vi "Move Distance in Constant Acceleration.vi"(7 "Time Between Points (ms)":dbl, 8 "Error In":errorcluster, 9 "Acceleration (in/s2)":dbl, 10 "Distance (in)":dbl, 11 "Initial Snapshot":T2) -> (0 "Error Out":errorcluster, 1 "Duration (s)":dbl, 2 "Motion Profile Portion":T1[](array[typedef]), 3 "Final Snapshot":T2)   [LabVIEW 2019, in "Motion Profile Generator.lvclass"]
uses:
  Motion Profile Generator.lvclass
  Type Defs/Motion Snapshot.ctl
  Type Defs/Motion Profile Point.ctl
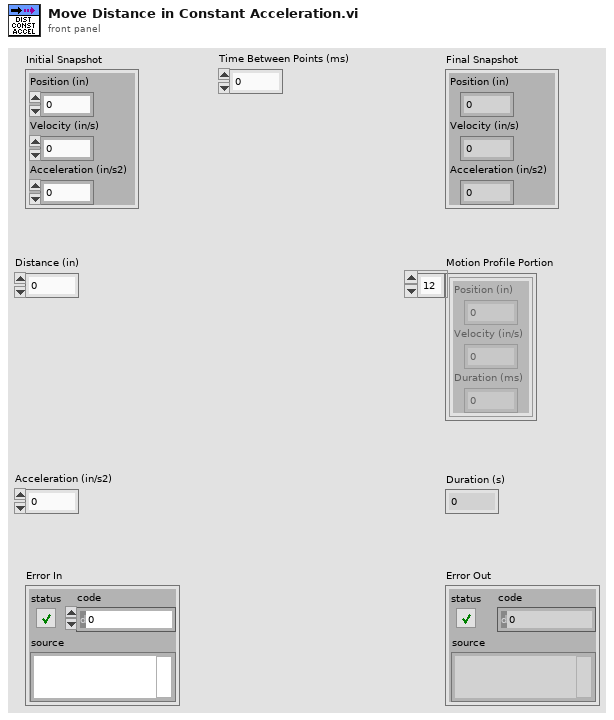
[diagram p1: front panel]
types:
  T1 = typedef "Motion Profile Generator.lvclass/Motion Profile Point.ctl" = cluster{"Position (in)":dbl, "Velocity (in/s)":dbl, "Duration (ms)":dbl}
  T2 = typedef "Motion Profile Generator.lvclass/Motion Snapshot.ctl" = cluster{"Position (in)":dbl, "Velocity (in/s)":dbl, "Acceleration (in/s2)":dbl}
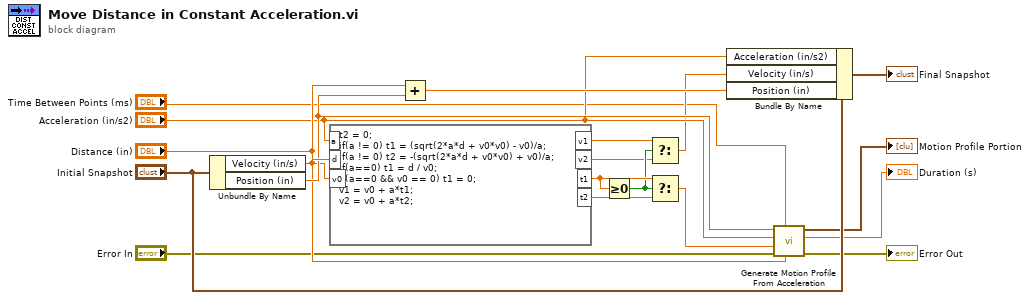
[diagram p0: block diagram]
diagram:
  n1 = Unbundle By Name("Initial Snapshot") -> ("Velocity (in/s)"=w11:dbl, "Position (in)"=w13:dbl)
  n2 = formula code="t2 = 0;\nif(a != 0) t1 = (sqrt(2*a*d + v0*v0) - v0)/a;\nif(a != 0) t2 = -(sqrt(2*a*d + v0*v0) + v0)/a;\nif(a==0) t1 = d / v0;\nif(a==0 && v0 == 0) t1 = 0;\nv1 = v0 + a*t1;\nv2 = v0 + a*t2;"("a"="Acceleration (in/s2)", "d"="Distance (in)", "v0"=w11) -> ("t1"=w6:dbl, "v1"=w4:dbl, "t2"=w7:dbl, "v2"=w3:dbl)
  n3 = Add(x="Distance (in)", y=w13) -> (x+y=w17:dbl)
  n4 = Greater Or Equal To 0?(x=w6) -> (x >= 0?=w5:bool)
  n5 = Select(t=w4, s=w5, f=w3) -> (s? t:f=w2:dbl)
  n6 = Select(t=w6, s=w5, f=w7) -> (s? t:f=w8:dbl)
  n7 = Bundle By Name(cluster="Initial Snapshot", "Acceleration (in/s2)"="Acceleration (in/s2)", "Velocity (in/s)"=w2, "Position (in)"=w17) -> (→"Final Snapshot":T2)
  n8 = call "Generate Motion Profile From Acceleration.vi"("Initial Velocity (in/s)"=w11, "Time Between Points (ms)"="Time Between Points (ms)", "Error In"="Error In", "Movement Duration (s)"=w8, "Acceleration (in/s2)"="Acceleration (in/s2)", "Initial Position (in)"=w13) -> ("Error Out"=→"Error Out":errorcluster, "Duration (s)"=→"Duration (s)":dbl, "Motion Profile Portion"=→"Motion Profile Portion":T1[])  [unwired: 3 in]
